vi "写入单个寄存器 (子VI).vi"(9 "值":u16, 10 "address":u16, 11 "VISA引用句柄输入":refnum<visa-resource-name>) -> ()   [LabVIEW 2016, in "斯坦道CODMn.lvlib"]
uses:
  <vilib>/Plasmionique/MB Master/MB_Master_Serial/MB_Master_Serial.lvclass
  F:/Program Files/National Instruments/LabVIEW 2016/vi.lib/Plasmionique/MB Master/MB_Master/MB_Master.lvclass
  <vilib>/Plasmionique/MB Master/MB Master.lvlib
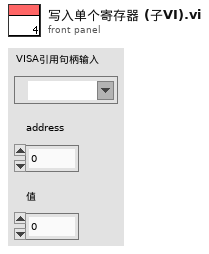
[diagram p1: front panel]
types:
  T1 = cluster{"baud rate (bps)":u32, "stop bits":u16, "parity":u16, "flow control":u16, "timeout":u32, "retries":i32}
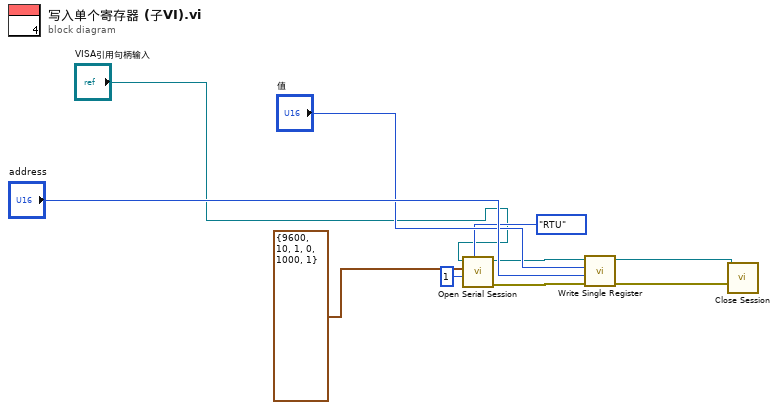
[diagram p0: block diagram]
diagram:
  n1 = call <vilib>:"Open Serial Session.vi"("Mode (RTU)"=enum16{"RTU", "ASCII"}."RTU", "Slave ID"=u8 1, "Serial Config"=T1 {"baud rate (bps)"=9600, "stop bits"=10, "parity"=1, "flow control"=0, "timeout"=1000, "retries"=1}, "VISA Resource"="VISA引用句柄输入") -> ("Error out"=w8:errorcluster, "MB_Serial session"=w5:refnum<class "MB_Master_Serial.lvclass">)  [unwired: 6 in]
  n2 = call <vilib>:"Write Single Register.vi"("error in (no error)"=w8, "value"="address", "address"="值", "MB session in"=w5) -> ("error out"=w9:errorcluster, "MB session out"=w10:refnum<class "MB_Master_Serial.lvclass">)  [unwired: 6 in]
  n3 = call-dynamic "Close Session.vi"("error in (no error)"=w9, "MB_Serial session"=w10) -> ()  [unwired: 9 in, 1 out]
